vi "JSON_Unescape.vi"(7 "error in (no error)":errorcluster, 9 "String In":string) -> (0 "error out":errorcluster, 2 "Unescaped String Out":string)   [LabVIEW 2011, in "JSON Value.lvclass"]
doc: "Removes reverse obliques (escapes) from the <b>Strin In</b> text and strips off the the leading and trailing quotes and square brackets.\nSupports the following escape characters:\n\\\"\n \\'\n \\[\n\\]\n\\{\n\\}\n\\\\"
uses:
  JSON Value.lvclass
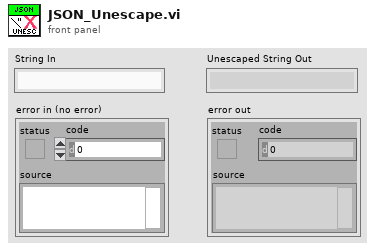
[diagram p1: front panel]
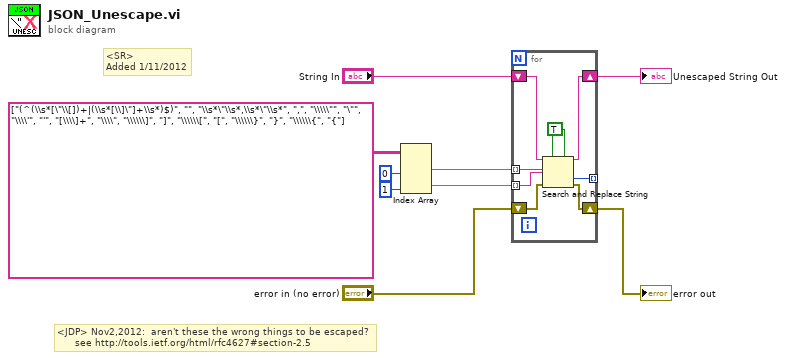
[diagram p0: block diagram]
diagram:
  # "<JDP> Nov2,2012:  aren't these the wrong things to be escaped?\n      see http://tools.ietf.org/html/rfc4627#section-2.5"
  # "<SR>\nAdded 1/11/2012"
  n1 = Index Array(array=string[][] [["(^(\\s*[\"\\[])+|(\\s*[\\]\"]+\\s*)$)", ""], ["\\s*\"\\s*,\\s*\"\\s*", ","], ["\\\\\"", "\""], ["\\\\'", "'"], ["[\\\\]+", "\\\\"], ["\\\\\\]", "]"], ["\\\\\\[", "["], ["\\\\\\}", "}"], ["\\\\\\{", "{"]], index (col) #1=0 ("disabled index (col)"), index (col) #2=1 ("index (col)")) -> (element #1=w6:string[], element #2=w5:string[])  [unwired: 2 in]
  n2 = for {
    tunnel: w6 -> [w15] mode=indexing
    tunnel: w5 -> [w14] mode=indexing
    shift-right: [w16] -> w3
    shift-left: "String In" -> [w17]
    tunnel: [w13] -> _ mode=indexing
    shift-right: [w11] -> w1
    shift-left: "error in (no error)" -> [w12]
    w10 = TRUE ("replace all? (F)")
    n3 = Search and Replace String(replace all?=w10, multiline?=w10, input string=w17, search string=w15, replace string=w14, error in=w12) -> (result string=w16:string, offset past replacement=w13:i32, error out=w11:errorcluster)  [unwired: 2 in, 1 out]
  }
  "Unescaped String Out" <- w3
  "error out" <- w1
